vi "VCO.vi"(9 "M":fxp<+,32,32>) -> (1 "Sine Sample":fxp<+/-,8,8>)   [LabVIEW 2015]
doc: "Emulates traditional VCO modules.\nIt outputs a single sample of a sine waveform every clock cycle.\nAs it uses DDS generation, a phase increment, represented by 'M', must be specified. Almost every audio frequency can be obtained, with a maximum resolution of 0.01 Hz, by applying the equation:\n\n Fout = M*Fclk / (2^32)"
uses:
  <vilib>/rvi/IPIntegrationNode/IPINode_Typedef/niFpgaIPINodeSupportedFamilies.ctl
  <vilib>/rvi/IPIntegrationNode/IPINode_Utilities/niFpgaIPINodeSimCore.vi
  <vilib>/rvi/XilinxIP/XIPIN_XNode/niFpgaXIPIN.xnode
  OSC/Xilinx DDS Compiler/xsim.dir/Xilinx_DDS_Compiler_8613DEDBA1A240988A97A4484D154CDC/xsimk_8613DEDBA1A240988A97A4484D154CDC.dll
  <vilib>/rvi/IPIntegrationNode/IPINode_Xnode/niFpgaIPINode.xnode
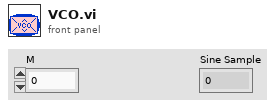
[diagram p1: front panel]
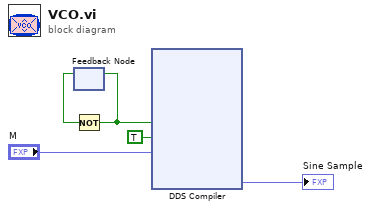
[diagram p0: block diagram]
diagram:
  n1 = feedback #1() -> (w4:bool)  [unwired: 1 in]
  n2 = Not(x=w4) -> (.not. x?=w1:bool)
  n3 = feedback-in #1(w1) -> ()
  n4 = xnode ("DDS Compiler")("aclk"=w1, "s_axis_config_tvalid"=TRUE, "s_axis_config_tdata"="M") -> ("m_axis_data_tdata"=→"Sine Sample":fxp<+/-,8,8>)  [unwired: 1 out]
